vi "1A Interpret NMEA Sentence.vi"(11 "NMEA Sentence":string) -> ()   [LabVIEW 2011]
doc: "Interprets the NMEA 0813 sentences that we are using from our Airmar PB200 WeatherStation sensor.\nBy Jaime McCandless\nTODO: finish implementing NMEA sentences"
uses:
  2-Think/2 Typedefs/Velocity.ctl
  2-Think/2 Typedefs/apparent wind.ctl
  2-Think/2 Typedefs/pitch and roll.ctl
  2-Think/2 Globals/2 Global.vi
  <vilib>/regexp/Match Regular Expression.xnode
panel:
  out "Meteorological Data":T1
  in  "UTC Time Zone":i32=-5
  out "Tab Control":T2(tab)
  out "GPS (GGA) Data":T3
  out "GPS (GLL) Data":T4
  out "UTC Time":timestamp
  out "Local Time":timestamp
  out "Lattitude (ddmm.mmmm)":dbl format="%_8g"
  out "Lattitude North/South":string
  out "Longitude (ddmm.mmmm)":dbl format="%_8g"
  out "Longitude East/West":string
  out "Speed over ground (knots)":dbl format="%_3g"
  out "Course over ground (degrees)":dbl format="%_4g"
  out "Magnetic Variation (degrees)":dbl format="%_4g"
  out "Variation East/West":string
  out "GPS (RMC) Data":T5 {"Course over ground (degrees)" format="%#.6g"; "Speed over ground (knots)" format="%#.6g"; "Magnetic Variation (degrees)" format="%#.6g"; "Longitude (ddmm.mmmm)" format="%#.6g"; "Lattitude (ddmm.mmmm)" format="%#.6g"}
  out "GPS Data Valid?":bool
  out "GPS (VTG) Data":T6
  out "Heading":dbl
  out "Turn (ROT) Data":T7
  out "Wind (MWV) Data":T8
  out "Transducer (XDR) B Data":cluster{"Pitch (deg)":dbl, "Roll (deg)":dbl}
  out "Transducer (XDR) A Data":T9
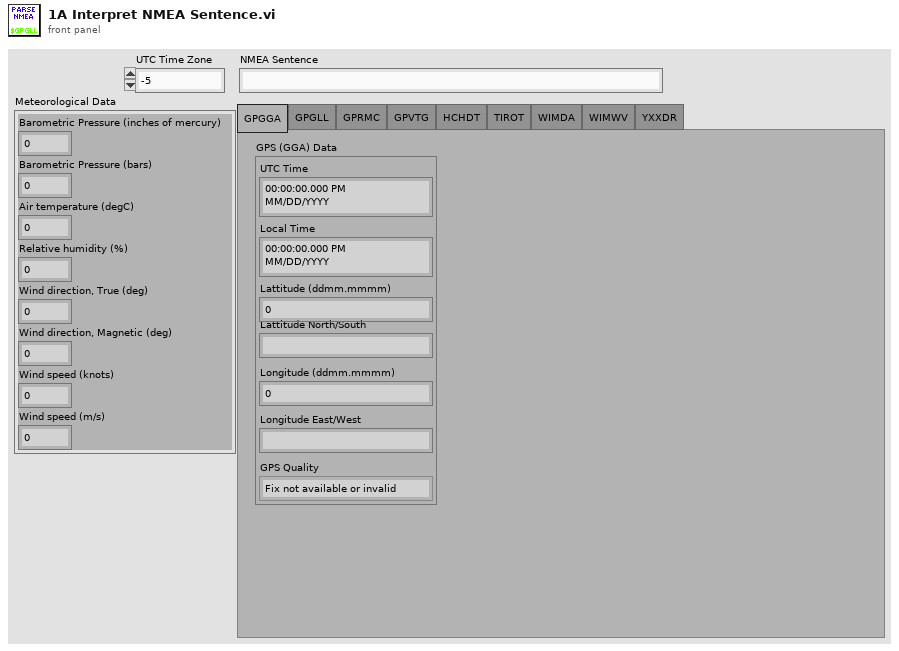
[diagram p1: front panel]
types:
  T1 = cluster{"Barometric Pressure (inches of mercury)":dbl, "Barometric Pressure (bars)":dbl, "Air temperature (degC)":dbl, "Relative humidity (%)":dbl, "Wind direction, True (deg)":dbl, "Wind direction, Magnetic (deg)":dbl, "Wind speed (knots)":dbl, "Wind speed (m/s)":dbl}
  T2 = enum32{"GPGGA", "GPGLL", "GPRMC", "GPVTG", "HCHDT", "TIROT", "WIMDA", "WIMWV", "YXXDR"}
  T3 = cluster{"UTC Time":timestamp, "Local Time":timestamp, "Lattitude (ddmm.mmmm)":dbl, "Lattitude North/South":string, "Longitude (ddmm.mmmm)":dbl, "Longitude East/West":string, "GPS Quality":enum16{"Fix not available or invalid", "GPS SPS Mode, fix valid", "Differential GPS, SPS Mode, fix valid", "GPS PPS Mode, fix valid", "Real Time Kinematic (RTK)", "Float RTK", "Estimated (dead reckoning) Mode", "Manual Input Mode", "Simulator Mode"}}
  T4 = cluster{"UTC Time":timestamp, "Local Time":timestamp, "Lattitude (ddmm.mmmm)":dbl, "Lattitude North/South":string, "Longitude (ddmm.mmmm)":dbl, "Longitude East/West":string, "GPS Mode":string, "GPS Data Valid?":bool}
  T5 = cluster{"UTC Time":timestamp, "Local Time":timestamp, "Lattitude (ddmm.mmmm)":dbl, "Lattitude North/South":string, "Longitude (ddmm.mmmm)":dbl, "Longitude East/West":string, "Magnetic Variation (degrees)":dbl, "Variation East/West":string, "Speed over ground (knots)":dbl, "Course over ground (degrees)":dbl}
  T6 = cluster{"Course Over Ground (True)":dbl, "Course Over Ground (Magnetic)":dbl, "Speed Over Ground (Knots)":dbl, "Speed Over Ground (km/hr)":dbl, "GPS Mode":string}
  T7 = cluster{"Rate of Turn (deg/min)":dbl, "Turn Rotation Data Valid?":bool}
  T8 = cluster{"Angle relative to boat (deg)":dbl, "Wind Data Valid?":bool, "Wind speed (knots)":dbl, "True (T) or Relative (R)":string}
  T9 = cluster{"Calc. Relative Wind Chill (degC)":dbl, "Calc. Theoretical Wind Chill (degC)":dbl, "Calc. Heat Index (degC)":dbl, "Meas. Barometric Pressure (bars)":dbl}
  T10 = cluster{"second":i32, "minute":i32, "hour":i32, "day of month":i32, "month":i32, "year":i32, "day of week":i32, "day of year":i32, "is DST":i32}
  T11 = typedef "Velocity.ctl" = cluster{"East":dbl, "North":dbl}
  T12 = typedef "apparent wind.ctl" = cluster{"Toward Fore":dbl, "Toward Starboard":dbl}
  T13 = typedef "pitch and roll.ctl" = cluster{"Pitch":dbl, "Roll":dbl}
  T14 = typedef "UTM Location.ctl" = cluster{"UTM Zone":dbl, "Hemisphere":enum16{"North", "South"}, "East":dbl, "North":dbl}
  T15 = typedef "generalized sensor status.ctl" = cluster{"Sensor Connected":T16, "Sensor Initialized":T16, "Sensor OK":T16, "Latest Error String":string, "GPS Lock":T16}
  T16 = typedef "indicator LED.ctl" = bool
  T17 = typedef "robot velocity.ctl" = cluster{"East":dbl, "North":dbl}
  T18 = typedef "heading.ctl" = dbl
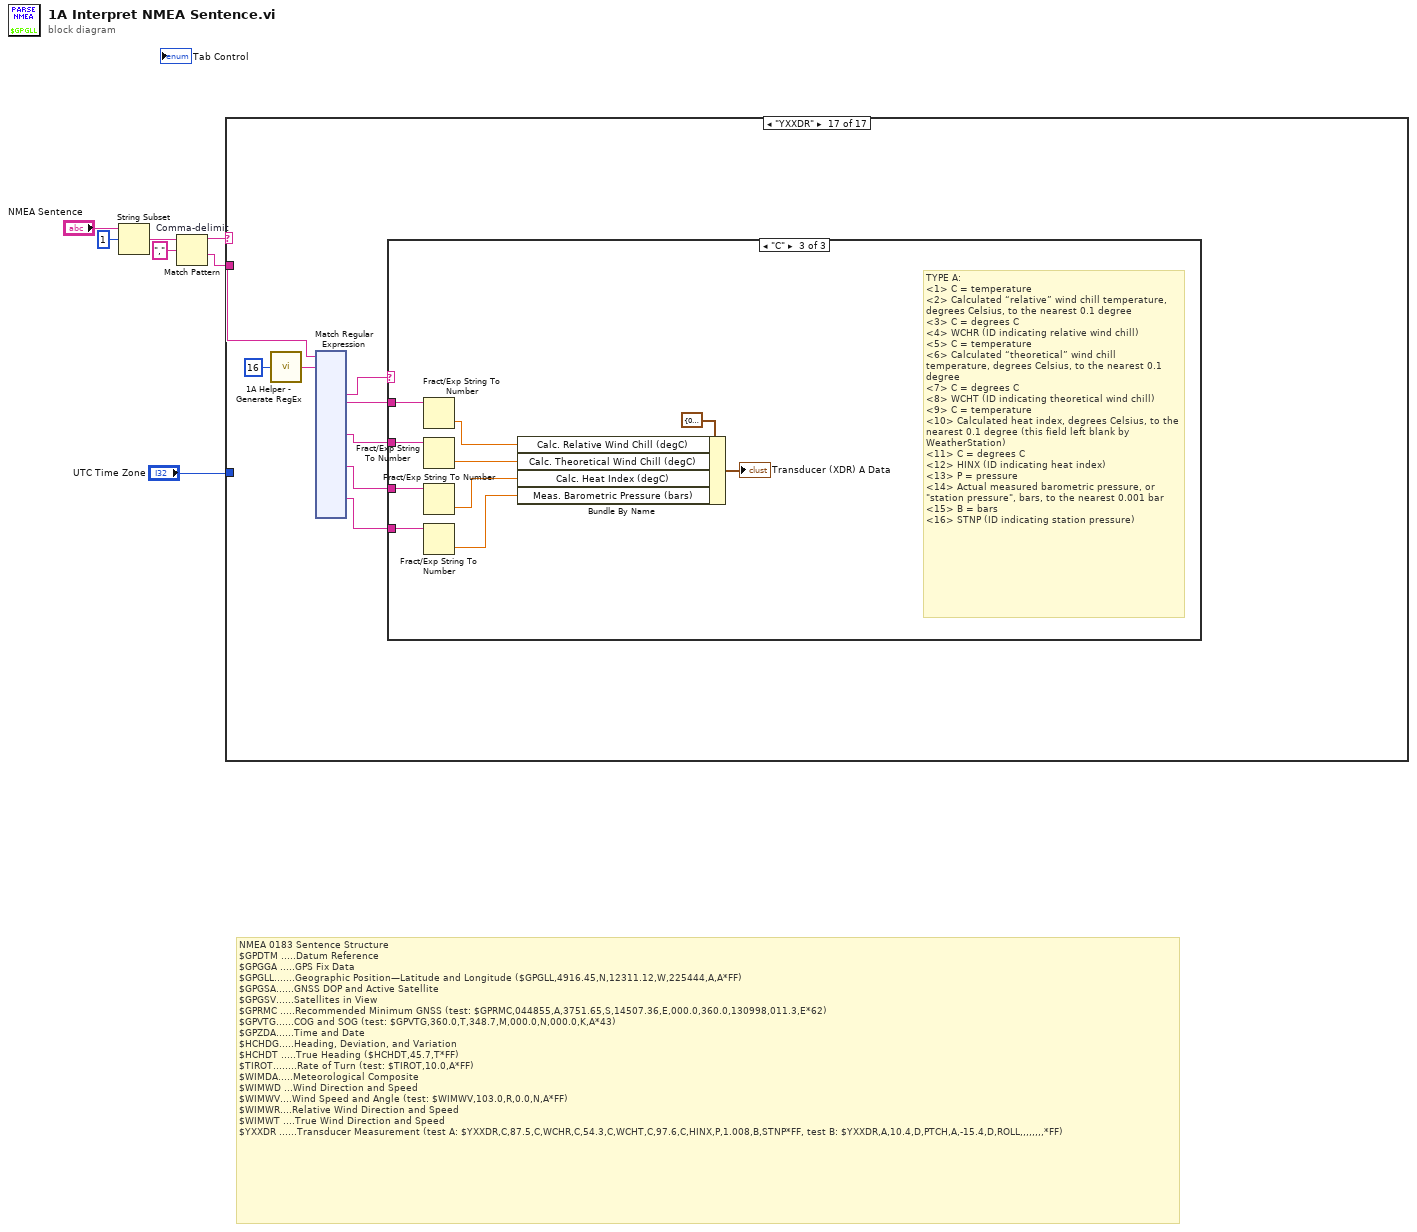
[diagram p0: block diagram]
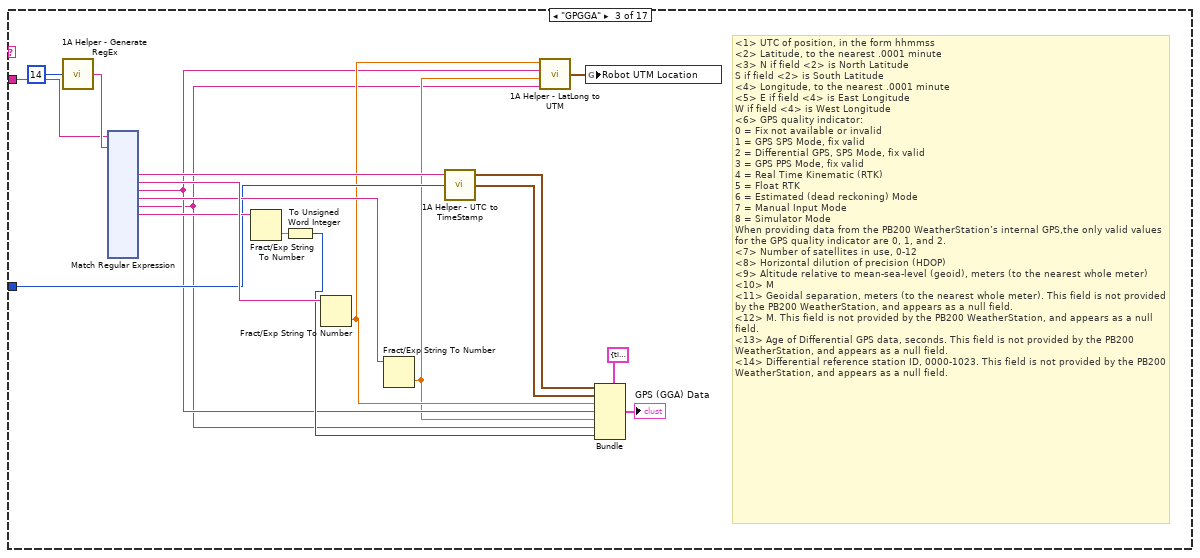
[diagram p4: hidden frame]
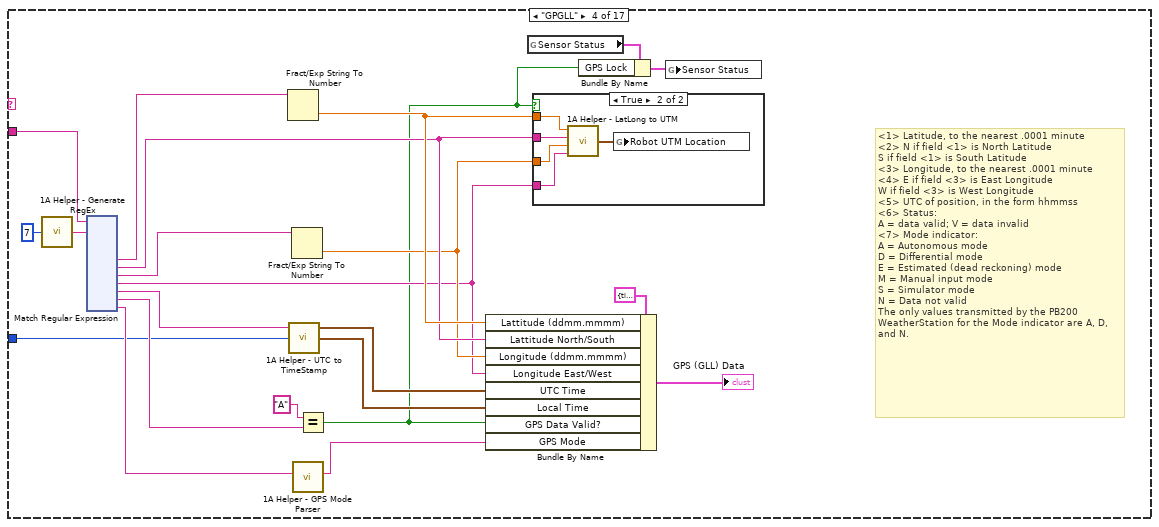
[diagram p5: hidden frame]
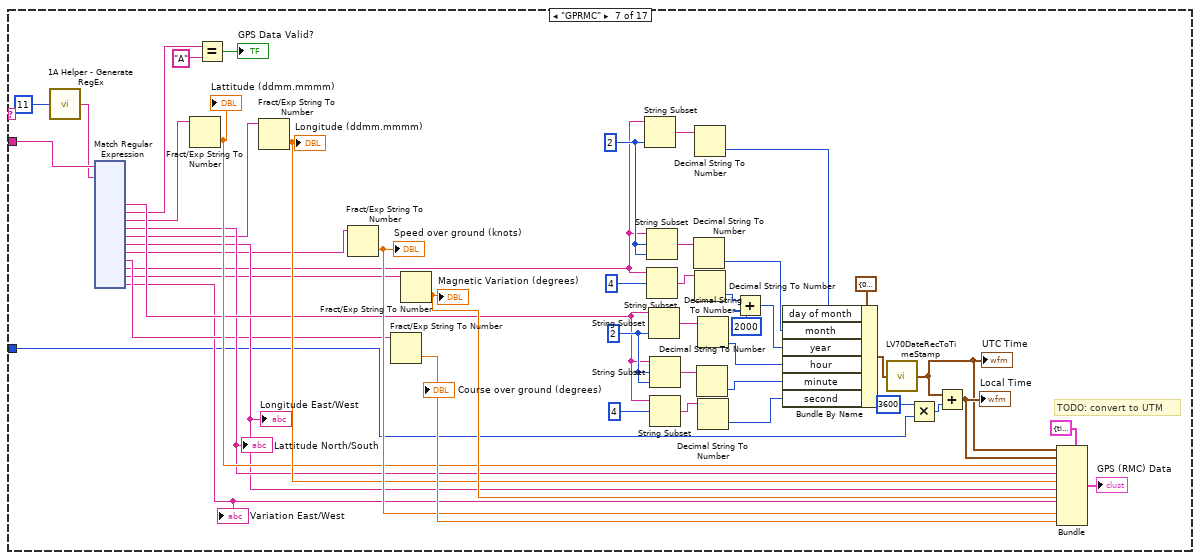
[diagram p9: hidden frame]
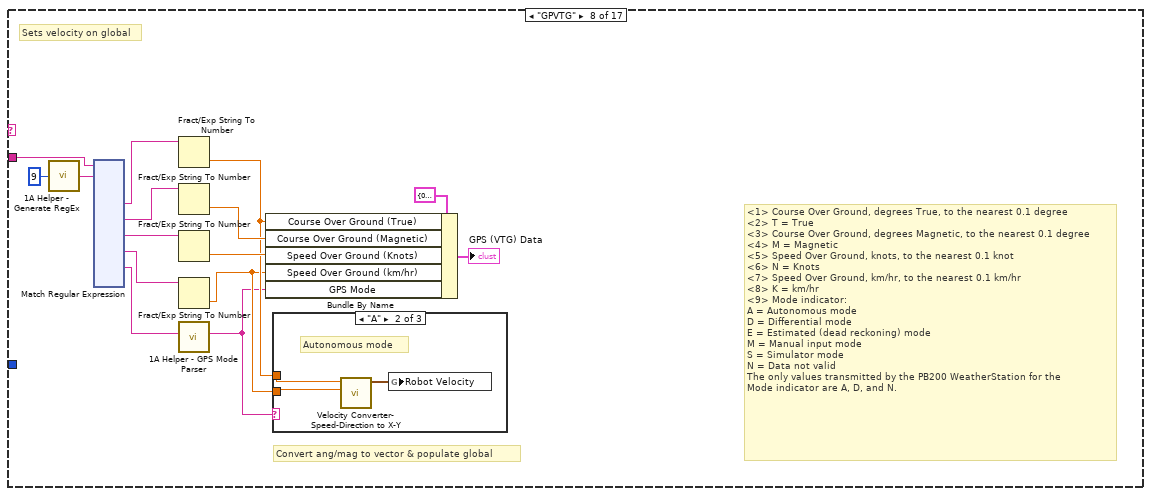
[diagram p10: hidden frame]
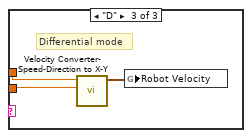
[diagram p12: hidden frame]
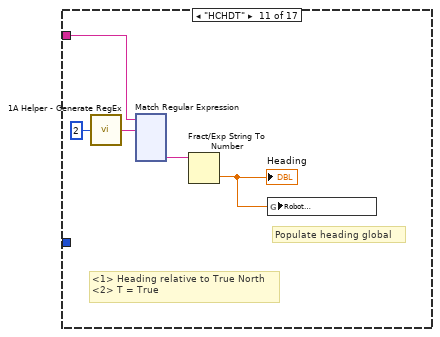
[diagram p15: hidden frame]
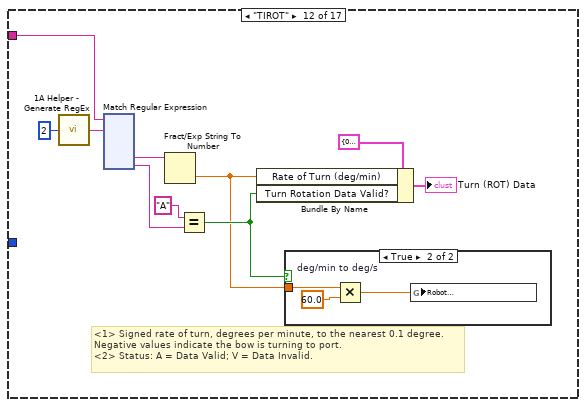
[diagram p16: hidden frame]
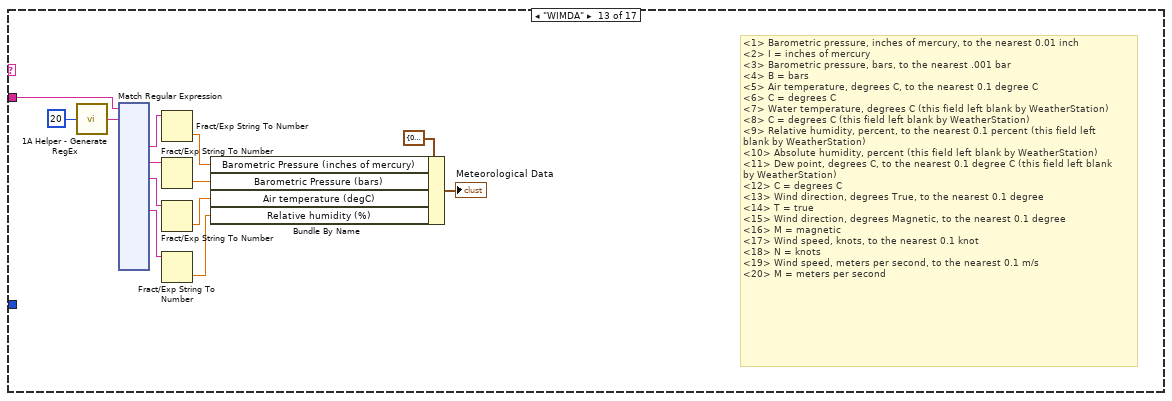
[diagram p18: hidden frame]
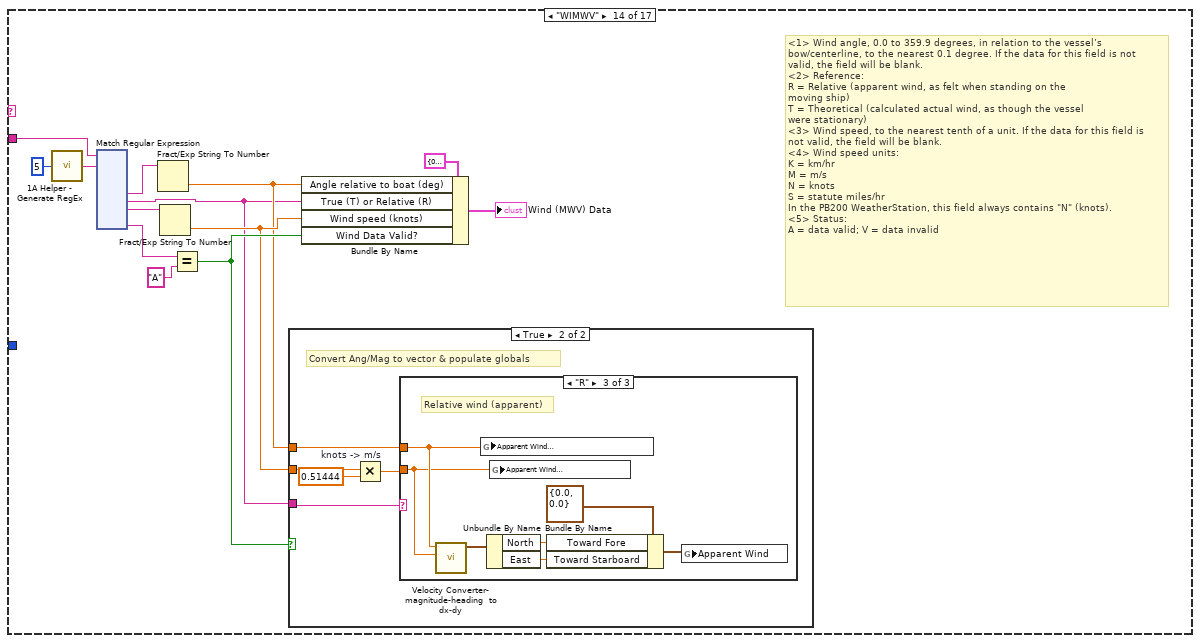
[diagram p19: hidden frame]
diagram:
  # "NMEA 0183 Sentence Structure\n$GPDTM .....Datum Reference\n$GPGGA .....GPS Fix Data\n$GPGLL.......Geographic Position—Latitude and Longitude ($GPGLL,4916.45,N,12311.12,W,225444,A,A*FF)\n$GPGSA......GNSS DOP and Active Satellite\n$GPGSV......Satellites in View\n$GPRMC .....Recommended Minimum GNSS (test: $GPRMC,044855,A,3751.65,S,14507.36,E,000.0,360.0,130998,011.3,E*62)\n$GPVTG......COG and SOG (test: $GPVTG,360.0,T,348.7,M,000.0,N,000.0,K,A*43)\n$GPZDA......Time and Date\n$HCHDG.....Heading, Deviation, and Variation\n$HCHDT .....True Heading ($HCHDT,45.7,T*FF)\n$TIROT........Rate of Turn (test: $TIROT,10.0,A*FF)\n$WIMDA.....Meteorological Composite\n$WIMWD ...Wind Direction and Speed\n$WIMWV....Wind Speed and Angle (test: $WIMWV,103.0,R,0.0,N,A*FF)\n$WIMWR....Relative Wind Direction and Speed\n$WIMWT ....True Wind Direction and Speed\n$YXXDR ......Transducer Measurement (test A: $YXXDR,C,87.5,C,WCHR,C,54.3,C,WCHT,C,97.6,C,HINX,P,1.008,B,STNP*FF, test B: $YXXDR,A,10.4,D,PTCH,A,-15.4,D,ROLL,,,,,,,,*FF)"
  n1 = String Subset(string="NMEA Sentence", offset (0)=1) -> (substring=w4:string)  [unwired: 1 in]
  n2 = Match Pattern "Comma-delimit"(string=w4, regular expression=",") -> (before substring=w5:string, after substring=w6:string)  [unwired: 1 in, 2 out]
  n3 = case shown="\"YXXDR\"" w5 {
    tunnel: w6 -> [_ _ w24 w166 _ _ w310 w479 _ _ w613 w735 w866 w1005 _ _ w1153]
    tunnel: "UTC Time Zone" -> [_ _ w13 w158 _ _ w296 _ _ _ _ _ _ _ _ _ _]
    frame "", Default {
    }
    frame "GPDTM" {
      # "unimplemented"
    }
    frame "GPGGA" {
      # "<1> UTC of position, in the form hhmmss\n<2> Latitude, to the nearest .0001 minute\n<3> N if field <2> is North Latitude\nS if field <2> is South Latitude\n<4> Longitude, to the nearest .0001 minute\n<5> E if field <4> is East Longitude\nW if field <4> is West Longitude\n<6> GPS quality indicator:\n0 = Fix not available or invalid\n1 = GPS SPS Mode, fix valid\n2 = Differential GPS, SPS Mode, fix valid\n3 = GPS PPS Mode, fix valid\n4 = Real Time Kinematic (RTK)\n5 = Float RTK\n6 = Estimated (dead reckoning) Mode\n7 = Manual Input Mode\n8 = Simulator Mode\nWhen providing data from the PB200 WeatherStation’s internal GPS,the only valid values for the GPS quality indicator are 0, 1, and 2.\n<7> Number of satellites in use, 0-12\n<8> Horizontal dilution of precision (HDOP)\n<9> Altitude relative to mean-sea-level (geoid), meters (to the nearest whole meter)\n<10> M\n<11> Geoidal separation, meters (to the nearest whole meter). This field is not provided by the PB200 WeatherStation, and appears as a null field.\n<12> M. This field is not provided by the PB200 WeatherStation, and appears as a null field.\n<13> Age of Differential GPS data, seconds. This field is not provided by the PB200 WeatherStation, and appears as a null field.\n<14> Differential reference station ID, 0000-1023. This field is not provided by the PB200 WeatherStation, and appears as a null field."
      n4 = call "1A Helper - Generate RegEx.vi"("# Datums"=14) -> ("RegEx"=w25:string)
      n5 = xnode "Match Regular Expression"("input string"=w24, "regular expression"=w25) -> ("submatch 1"=w16:string, "submatch 2"=w22:string, "submatch 3"=w10:string, "submatch 4"=w21:string, "submatch 5"=w8:string, "submatch 6"=w20:string)  [unwired: 4 in, 10 out]
      n6 = Fract/Exp String To Number(string=w20) -> (number=w19:dbl)  [unwired: 3 in, 1 out]
      n7 = To Unsigned Word Integer(number=w19) -> (unsigned 16bit integer=w18:u16)
      n8 = Fract/Exp String To Number(string=w22) -> (number=w11:dbl)  [unwired: 3 in, 1 out]
      n9 = Fract/Exp String To Number(string=w21) -> (number=w9:dbl)  [unwired: 3 in, 1 out]
      n10 = call "1A Helper - UTC to TimeStamp.vi"("UTC Time Zone in"=w13, "UTC (hhmmss)"=w16) -> ("Local Time"=w14:timestamp, "UTC Time"=w15:timestamp)  [unwired: 2 in]
      n11 = call "1A Helper - LatLong to UTM.vi"("East/West"=w8, "Longitude"=w9, "North/South"=w10, "Latitude"=w11) -> ("Robot UTM Location"=w12:T14)
      n12 = global write "2 Global.vi" "Robot UTM Location"(w12) -> ()
      n13 = Bundle(cluster=T3 {"UTC Time"=timestamp(0 s since 1904-01-01), "Local Time"=timestamp(0 s since 1904-01-01), "Lattitude (ddmm.mmmm)"=0.0, "Lattitude North/South"="", "Longitude (ddmm.mmmm)"=0.0, "Longitude East/West"="", "GPS Quality"=enum."GPS SPS Mode, fix valid"} ("Cluster"), "UTC Time"=w15, "Local Time"=w14, "Lattitude (ddmm.mmmm)"=w11, "Lattitude North/South"=w10, "Longitude (ddmm.mmmm)"=w9, "Longitude East/West"=w8, "GPS Quality"=w18) -> (→"GPS (GGA) Data":T3)
    }
    frame "GPGLL" {
      # "<1> Latitude, to the nearest .0001 minute\n<2> N if field <1> is North Latitude\nS if field <1> is South Latitude\n<3> Longitude, to the nearest .0001 minute\n<4> E if field <3> is East Longitude\nW if field <3> is West Longitude\n<5> UTC of position, in the form hhmmss\n<6> Status:\nA = data valid; V = data invalid\n<7> Mode indicator:\nA = Autonomous mode\nD = Differential mode\nE = Estimated (dead reckoning) mode\nM = Manual input mode\nS = Simulator mode\nN = Data not valid\nThe only values transmitted by the PB200 WeatherStation for the Mode indicator are A, D, and N."
      n14 = call "1A Helper - Generate RegEx.vi"("# Datums"=7) -> ("RegEx"=w170:string)
      n15 = xnode "Match Regular Expression"("input string"=w166, "regular expression"=w170) -> ("submatch 1"=w169:string, "submatch 2"=w155:string, "submatch 3"=w168:string, "submatch 4"=w153:string, "submatch 5"=w165:string, "submatch 6"=w161:string, "submatch 7"=w167:string)  [unwired: 4 in, 5 out]
      n16 = Fract/Exp String To Number(string=w169) -> (number=w156:dbl)  [unwired: 3 in, 1 out]
      n17 = call "1A Helper - UTC to TimeStamp.vi"("UTC Time Zone in"=w158, "UTC (hhmmss)"=w165) -> ("Local Time"=w160:timestamp, "UTC Time"=w159:timestamp)  [unwired: 2 in]
      n18 = Fract/Exp String To Number(string=w168) -> (number=w154:dbl)  [unwired: 3 in, 1 out]
      n19 = call "1A Helper - GPS Mode Parser.vi"("GPS Mode (Char)"=w167) -> ("GPS Mode (Description)"=w163:string)  [unwired: 6 in]
      n20 = Equal?(x="A" ("y"), y=w161) -> (x = y?=w150:bool)
      n21 = Bundle By Name(cluster=T4 {"UTC Time"=timestamp(0 s since 1904-01-01), "Local Time"=timestamp(0 s since 1904-01-01), "Lattitude (ddmm.mmmm)"=0.0, "Lattitude North/South"="", "Longitude (ddmm.mmmm)"=0.0, "Longitude East/West"="", "GPS Mode"="", "GPS Data Valid?"=FALSE} ("Cluster"), "Lattitude (ddmm.mmmm)"=w156, "Lattitude North/South"=w155, "Longitude (ddmm.mmmm)"=w154, "Longitude East/West"=w153, "UTC Time"=w159, "Local Time"=w160, "GPS Data Valid?"=w150, "GPS Mode"=w163) -> (→"GPS (GLL) Data":T4)
      n22 = global read "2 Global.vi" "Sensor Status"() -> (w151:T15)
      n23 = case shown="True" w150 {
        tunnel: w156 -> [_ w176]
        tunnel: w155 -> [_ w175]
        tunnel: w154 -> [_ w174]
        tunnel: w153 -> [_ w173]
        frame False {
        }
        frame True {
          n24 = call "1A Helper - LatLong to UTM.vi"("East/West"=w173, "Longitude"=w174, "North/South"=w175, "Latitude"=w176) -> ("Robot UTM Location"=w172:T14)
          n25 = global write "2 Global.vi" "Robot UTM Location"(w172) -> ()
        }
      }
      n26 = Bundle By Name(cluster=w151, "GPS Lock"=w150) -> (w152:T15)
      n27 = global write "2 Global.vi" "Sensor Status"(w152) -> ()
    }
    frame "GPGSA" {
      # "unimplemented"
    }
    frame "GPGSV" {
      # "unimplemented"
    }
    frame "GPRMC" {
      w328 = 2 ("length (rest)")
      w318 = 2 ("length (rest)")
      # "TODO: convert to UTM"
      n28 = call "1A Helper - Generate RegEx.vi"("# Datums"=11) -> ("RegEx"=w298:string)
      n29 = xnode "Match Regular Expression"("input string"=w310, "regular expression"=w298) -> ("submatch 1"=w309:string, "submatch 2"=w308:string, "submatch 3"=w307:string, "submatch 4"=w306:string, "submatch 5"=w305:string, "submatch 6"=w304:string, "submatch 7"=w303:string, "submatch 8"=w302:string, "submatch 9"=w301:string, "submatch 10"=w300:string, "submatch 11"=w299:string)  [unwired: 4 in, 5 out]
      "Lattitude North/South" <- w306
      "Longitude East/West" <- w304
      "Variation East/West" <- w299
      n30 = Fract/Exp String To Number(string=w307) -> (number=w337:dbl)  [unwired: 3 in, 1 out]
      "Lattitude (ddmm.mmmm)" <- w337
      n31 = Equal?(x=w308, y="A") -> (x = y?=→"GPS Data Valid?":bool)
      n32 = Fract/Exp String To Number(string=w305) -> (number=w338:dbl)  [unwired: 3 in, 1 out]
      "Longitude (ddmm.mmmm)" <- w338
      n33 = Fract/Exp String To Number(string=w303) -> (number=w340:dbl)  [unwired: 3 in, 1 out]
      "Speed over ground (knots)" <- w340
      n34 = Fract/Exp String To Number(string=w302) -> (number=w341:dbl)  [unwired: 3 in, 1 out]
      "Course over ground (degrees)" <- w341
      n35 = Fract/Exp String To Number(string=w300) -> (number=w339:dbl)  [unwired: 3 in, 1 out]
      "Magnetic Variation (degrees)" <- w339
      n36 = String Subset(string=w301, length (rest)=w328) -> (substring=w329:string)  [unwired: 1 in]
      n37 = String Subset(string=w301, offset (0)=w328, length (rest)=w328) -> (substring=w327:string)
      n38 = String Subset(string=w301, offset (0)=4) -> (substring=w325:string)  [unwired: 1 in]
      n39 = String Subset(string=w309, length (rest)=w318) -> (substring=w314:string)  [unwired: 1 in]
      n40 = String Subset(string=w309, offset (0)=w318, length (rest)=w318) -> (substring=w320:string)
      n41 = String Subset(string=w309, offset (0)=4) -> (substring=w322:string)  [unwired: 1 in]
      n42 = Decimal String To Number(string=w327) -> (number=w331:i32)  [unwired: 2 in, 1 out]
      n43 = Decimal String To Number(string=w329) -> (number=w330:i32)  [unwired: 2 in, 1 out]
      n44 = Decimal String To Number(string=w325) -> (number=w332:i32)  [unwired: 2 in, 1 out]
      n45 = Decimal String To Number(string=w320) -> (number=w319:i32)  [unwired: 2 in, 1 out]
      n46 = Decimal String To Number(string=w314) -> (number=w317:i32)  [unwired: 2 in, 1 out]
      n47 = Decimal String To Number(string=w322) -> (number=w323:i32)  [unwired: 2 in, 1 out]
      n48 = Add(x=w332, y=2000) -> (x+y=w334:i32)
      n49 = Bundle By Name(cluster=T10 {"second"=0, "minute"=0, "hour"=0, "day of month"=0, "month"=0, "year"=0, "day of week"=0, "day of year"=0, "is DST"=0} ("date time rec"), "day of month"=w330, "month"=w331, "year"=w334, "hour"=w317, "minute"=w319, "second"=w323) -> (w315:T10)
      n50 = call <vilib>:"LV70DateRecToTimeStamp.vi"("date time rec"=w315) -> ("Time Stamp"=w335:timestamp)
      "UTC Time" <- w335
      n51 = Multiply(x=3600 ("number"), y=w296) -> (x*y=w297:i32)
      n52 = Add(x=w335, y=w297) -> (x+y=w336:timestamp)
      "Local Time" <- w336
      n53 = Bundle(cluster=T5 {"UTC Time"=timestamp(0 s since 1904-01-01), "Local Time"=timestamp(0 s since 1904-01-01), "Lattitude (ddmm.mmmm)"=0.0, "Lattitude North/South"="", "Longitude (ddmm.mmmm)"=0.0, "Longitude East/West"="", "Magnetic Variation (degrees)"=0.0, "Variation East/West"="", "Speed over ground (knots)"=0.0, "Course over ground (degrees)"=0.0} ("Cluster"), "UTC Time"=w335, "Local Time"=w336, "Lattitude (ddmm.mmmm)"=w337, "Lattitude North/South"=w306, "Longitude (ddmm.mmmm)"=w338, "Longitude East/West"=w304, "Magnetic Variation (degrees)"=w339, "Variation East/West"=w299, "Speed over ground (knots)"=w340, "Course over ground (degrees)"=w341) -> (→"GPS (RMC) Data":T5)
    }
    frame "GPVTG" {
      # "Convert ang/mag to vector & populate global"
      # "Sets velocity on global"
      # "<1> Course Over Ground, degrees True, to the nearest 0.1 degree\n<2> T = True\n<3> Course Over Ground, degrees Magnetic, to the nearest 0.1 degree\n<4> M = Magnetic\n<5> Speed Over Ground, knots, to the nearest 0.1 knot\n<6> N = Knots\n<7> Speed Over Ground, km/hr, to the nearest 0.1 km/hr\n<8> K = km/hr\n<9> Mode indicator:\nA = Autonomous mode\nD = Differential mode\nE = Estimated (dead reckoning) mode\nM = Manual input mode\nS = Simulator mode\nN = Data not valid\nThe only values transmitted by the PB200 WeatherStation for the\nMode indicator are A, D, and N."
      n54 = call "1A Helper - Generate RegEx.vi"("# Datums"=9) -> ("RegEx"=w480:string)
      n55 = xnode "Match Regular Expression"("input string"=w479, "regular expression"=w480) -> ("submatch 1"=w476:string, "submatch 3"=w475:string, "submatch 5"=w473:string, "submatch 7"=w471:string, "submatch 9"=w470:string)  [unwired: 4 in, 11 out]
      n56 = Fract/Exp String To Number(string=w476) -> (number=w469:dbl)  [unwired: 3 in, 1 out]
      n57 = Fract/Exp String To Number(string=w475) -> (number=w474:dbl)  [unwired: 3 in, 1 out]
      n58 = Fract/Exp String To Number(string=w473) -> (number=w472:dbl)  [unwired: 3 in, 1 out]
      n59 = Fract/Exp String To Number(string=w471) -> (number=w468:dbl)  [unwired: 3 in, 1 out]
      n60 = call "1A Helper - GPS Mode Parser.vi"("GPS Mode (Char)"=w470) -> ("GPS Mode (Description)"=w467:string)  [unwired: 6 in]
      n61 = Bundle By Name(cluster=T6 {"Course Over Ground (True)"=0.0, "Course Over Ground (Magnetic)"=0.0, "Speed Over Ground (Knots)"=0.0, "Speed Over Ground (km/hr)"=0.0, "GPS Mode"=""} ("GPS (VTG) Data 2"), "Course Over Ground (True)"=w469, "Course Over Ground (Magnetic)"=w474, "Speed Over Ground (Knots)"=w472, "Speed Over Ground (km/hr)"=w468, "GPS Mode"=w467) -> (→"GPS (VTG) Data":T6)
      n62 = case shown="\"A\"" w467 {
        tunnel: w469 -> [_ w482 w487]
        tunnel: w468 -> [_ w484 w486]
        frame "N", Default {
          # "Data not valid"
        }
        frame "A" {
          # "Autonomous mode"
          n63 = call "Velocity Converter- Speed-Direction to X-Y.vi"("Speed"=w484, "Heading"=w482) -> ("Robot Velocity Out"=w483:T17)  [unwired: 9 in]
          n64 = global write "2 Global.vi" "Robot Velocity"(w483) -> ()
        }
        frame "D" {
          # "Differential mode"
          n65 = call "Velocity Converter- Speed-Direction to X-Y.vi"("Speed"=w486, "Heading"=w487) -> ("Robot Velocity Out"=w485:T17)  [unwired: 9 in]
          n66 = global write "2 Global.vi" "Robot Velocity"(w485) -> ()
        }
      }
    }
    frame "GPZDA" {
      # "<1> UTC time of day, in the form hhmmss\n<2> UTC day, 01 to 31\n<3> UTC month, 01 to 12\n<4> UTC year (four digits, e.g. 2006)\n<5> Local time zone hours, 00 to +/-13 hrs\n<6> Local time zone minutes, 00 to +59"
    }
    frame "HCHDG " {
      # "<1> Magnetic sensor heading, degrees, to the nearest 0.1 degree.\n<2> Magnetic deviation, degrees east or west, to the nearest 0.1 degree.\n<3> E if field <2> is degrees East\nW if field <2> is degrees West\n<4> Magnetic variation, degrees east or west, to the nearest 0.1 degree.\n<5> E if field <4> is degrees East\nW if field <4> is degrees West"
    }
    frame "HCHDT" {
      # "Populate heading global"
      # "<1> Heading relative to True North\n<2> T = True"
      n67 = call "1A Helper - Generate RegEx.vi"("# Datums"=2) -> ("RegEx"=w614:string)
      n68 = xnode "Match Regular Expression"("input string"=w613, "regular expression"=w614) -> ("submatch 1"=w612:string)  [unwired: 4 in, 5 out]
      n69 = Fract/Exp String To Number(string=w612) -> (number=w611:dbl)  [unwired: 3 in, 1 out]
      "Heading" <- w611
      n70 = global write "2 Global.vi" "Robot\nHeading"(w611) -> ()
    }
    frame "TIROT" {
      # "<1> Signed rate of turn, degrees per minute, to the nearest 0.1 degree.\nNegative values indicate the bow is turning to port.\n<2> Status: A = Data Valid; V = Data Invalid."
      n71 = call "1A Helper - Generate RegEx.vi"("# Datums"=2) -> ("RegEx"=w737:string)
      n72 = xnode "Match Regular Expression"("input string"=w735, "regular expression"=w737) -> ("submatch 1"=w736:string, "submatch 2"=w731:string)  [unwired: 4 in, 5 out]
      n73 = Fract/Exp String To Number(string=w736) -> (number=w729:dbl)  [unwired: 3 in, 1 out]
      n74 = Equal?(x="A" ("y"), y=w731) -> (x = y?=w730:bool)
      n75 = Bundle By Name(cluster=T7 {"Rate of Turn (deg/min)"=0.0, "Turn Rotation Data Valid?"=TRUE} ("Turn (ROT) Data 2"), "Rate of Turn (deg/min)"=w729, "Turn Rotation Data Valid?"=w730) -> (→"Turn (ROT) Data":T7)
      n76 = case shown="True" w730 {
        tunnel: w729 -> [_ w740]
        frame False {
        }
        frame True {
          n77 = Multiply "deg/min to deg/s"(x=w740, y=60.0) -> (x*y=w741:dbl)
          n78 = global write "2 Global.vi" "Robot\nRate of Turn"(w741) -> ()
        }
      }
    }
    frame "WIMDA" {
      # "<1> Barometric pressure, inches of mercury, to the nearest 0.01 inch\n<2> I = inches of mercury\n<3> Barometric pressure, bars, to the nearest .001 bar\n<4> B = bars\n<5> Air temperature, degrees C, to the nearest 0.1 degree C\n<6> C = degrees C\n<7> Water temperature, degrees C (this field left blank by WeatherStation)\n<8> C = degrees C (this field left blank by WeatherStation)\n<9> Relative humidity, percent, to the nearest 0.1 percent (this field left\nblank by WeatherStation)\n<10> Absolute humidity, percent (this field left blank by WeatherStation)\n<11> Dew point, degrees C, to the nearest 0.1 degree C (this field left blank\nby WeatherStation)\n<12> C = degrees C\n<13> Wind direction, degrees True, to the nearest 0.1 degree\n<14> T = true\n<15> Wind direction, degrees Magnetic, to the nearest 0.1 degree\n<16> M = magnetic\n<17> Wind speed, knots, to the nearest 0.1 knot\n<18> N = knots\n<19> Wind speed, meters per second, to the nearest 0.1 m/s\n<20> M = meters per second"
      n79 = call "1A Helper - Generate RegEx.vi"("# Datums"=20) -> ("RegEx"=w867:string)
      n80 = xnode "Match Regular Expression"("input string"=w866, "regular expression"=w867) -> ("submatch 1"=w860:string, "submatch 3"=w859:string, "submatch 5"=w858:string, "submatch 9"=w857:string)  [unwired: 4 in, 17 out]
      n81 = Fract/Exp String To Number(string=w860) -> (number=w864:dbl)  [unwired: 3 in, 1 out]
      n82 = Fract/Exp String To Number(string=w859) -> (number=w863:dbl)  [unwired: 3 in, 1 out]
      n83 = Fract/Exp String To Number(string=w858) -> (number=w862:dbl)  [unwired: 3 in, 1 out]
      n84 = Fract/Exp String To Number(string=w857) -> (number=w861:dbl)  [unwired: 3 in, 1 out]
      n85 = Bundle By Name(cluster=T1 {"Barometric Pressure (inches of mercury)"=0.0, "Barometric Pressure (bars)"=0.0, "Air temperature (degC)"=0.0, "Relative humidity (%)"=0.0, "Wind direction, True (deg)"=0.0, "Wind direction, Magnetic (deg)"=0.0, "Wind speed (knots)"=0.0, "Wind speed (m/s)"=0.0} ("Meteorological Data"), "Barometric Pressure (inches of mercury)"=w864, "Barometric Pressure (bars)"=w863, "Air temperature (degC)"=w862, "Relative humidity (%)"=w861) -> (→"Meteorological Data":T1)
    }
    frame "WIMWV" {
      # "<1> Wind angle, 0.0 to 359.9 degrees, in relation to the vessel’s\nbow/centerline, to the nearest 0.1 degree. If the data for this field is not\nvalid, the field will be blank.\n<2> Reference:\nR = Relative (apparent wind, as felt when standing on the\nmoving ship)\nT = Theoretical (calculated actual wind, as though the vessel\nwere stationary)\n<3> Wind speed, to the nearest tenth of a unit. If the data for this field is\nnot valid, the field will be blank.\n<4> Wind speed units:\nK = km/hr\nM = m/s\nN = knots\nS = statute miles/hr\nIn the PB200 WeatherStation, this field always contains \"N\" (knots).\n<5> Status:\nA = data valid; V = data invalid"
      n86 = call "1A Helper - Generate RegEx.vi"("# Datums"=5) -> ("RegEx"=w1008:string)
      n87 = xnode "Match Regular Expression"("input string"=w1005, "regular expression"=w1008) -> ("submatch 1"=w1007:string, "submatch 2"=w997:string, "submatch 3"=w1002:string, "submatch 5"=w1001:string)  [unwired: 4 in, 6 out]
      n88 = Fract/Exp String To Number(string=w1007) -> (number=w998:dbl)  [unwired: 3 in, 1 out]
      n89 = Fract/Exp String To Number(string=w1002) -> (number=w999:dbl)  [unwired: 3 in, 1 out]
      n90 = Equal?(x=w1001, y="A") -> (x = y?=w1000:bool)
      n91 = case shown="True" w1000 {
        tunnel: w999 -> [_ w1011]
        tunnel: w998 -> [_ w1014]
        tunnel: w997 -> [_ w1013]
        frame False {
        }
        frame True {
          # "Convert Ang/Mag to vector & populate globals"
          n92 = Multiply "knots -> m/s"(x=w1011, y=0.51444) -> (x*y=w1012:dbl)
          n93 = case shown="\"R\"" w1013 {
            tunnel: w1012 -> [_ w1019 w1024]
            tunnel: w1014 -> [_ w1016 w1025]
            frame "", Default {
            }
            frame "T" {
              # "Theoretical wind (absolute)"
              n94 = global read "2 Global.vi" "Robot\nHeading"() -> (w1017:T18)
              n95 = Add "Get relative to compass, not boat"(x=w1017, y=w1016) -> (x+y=w1015:T18)
              n96 = call "Velocity Converter- magnitude-heading  to dx-dy.vi"("Magnitude"=w1019, "Heading"=w1015) -> ("Vector Out"=w1023:T11)  [unwired: 9 in]
              n97 = Unbundle By Name(w1023) -> ("North"=w1021:dbl, "East"=w1020:dbl)
              n98 = Bundle By Name(cluster=T11 {"East"=0.0, "North"=0.0} ("Absolute Wind"), "North"=w1021, "East"=w1020) -> (w1022:T11)
              n99 = global write "2 Global.vi" "Absolute Wind\nDirection (º)"(w1015) -> ()
              n100 = global write "2 Global.vi" "Absolute Wind\nSpeed"(w1019) -> ()
              n101 = global write "2 Global.vi" "Absolute Wind"(w1022) -> ()
            }
            frame "R" {
              # "Relative wind (apparent)"
              n102 = call "Velocity Converter- magnitude-heading  to dx-dy.vi"("Magnitude"=w1024, "Heading"=w1025) -> ("Vector Out"=w1026:T11)  [unwired: 9 in]
              n103 = global write "2 Global.vi" "Apparent Wind\nDirection (º)"(w1025) -> ()
              n104 = Unbundle By Name(w1026) -> ("North"=w1029:dbl, "East"=w1030:dbl)
              n105 = global write "2 Global.vi" "Apparent Wind\nSpeed"(w1024) -> ()
              n106 = Bundle By Name(cluster=T12 {"Toward Fore"=0.0, "Toward Starboard"=0.0} ("Apparent Wind"), "Toward Fore"=w1029, "Toward Starboard"=w1030) -> (w1028:T12)
              n107 = global write "2 Global.vi" "Apparent Wind"(w1028) -> ()
            }
          }
        }
      }
      n108 = Bundle By Name(cluster=T8 {"Angle relative to boat (deg)"=0.0, "Wind Data Valid?"=TRUE, "Wind speed (knots)"=0.0, "True (T) or Relative (R)"=""} ("Wind (MWV) Data 2"), "Angle relative to boat (deg)"=w998, "True (T) or Relative (R)"=w997, "Wind speed (knots)"=w999, "Wind Data Valid?"=w1000) -> (→"Wind (MWV) Data":T8)
    }
    frame "WIMWR" {
    }
    frame "WIMWT" {
    }
    frame "YXXDR" {
      n109 = call "1A Helper - Generate RegEx.vi"("# Datums"=16) -> ("RegEx"=w1155:string)
      n110 = xnode "Match Regular Expression"("input string"=w1153, "regular expression"=w1155) -> ("submatch 1"=w1152:string, "submatch 2"=w1151:string, "submatch 6"=w1150:string, "submatch 10"=w1149:string, "submatch 14"=w1148:string)  [unwired: 4 in, 16 out]
      n111 = case shown="\"C\"" w1152 {
        tunnel: w1151 -> [_ w1161 w1171]
        tunnel: w1150 -> [_ w1160 w1170]
        tunnel: w1149 -> [_ _ w1168]
        tunnel: w1148 -> [_ _ w1169]
        frame "", Default {
        }
        frame "A" {
          # "TYPE B:\n<1> A = angular displacement\n<2> Pitch: oscillation of vessel about its latitudinal axis. Bow moving up is positive. Value reported to the nearest 0.1 degree.\n<3> D = degrees\n<4> PTCH (ID indicating pitch of vessel)\n<5> A = angular displacement\n<6> Roll: oscillation of vessel about its longitudinal axis. Roll to the starboard is positive. Value reported to the nearest 0.1 degree.\n<7> D = degrees\n<8> ROLL (ID indicating roll of vessel)\n<9> Not used\n<10> Not used\n<11> Not used\n<12> Not used\n<13> Not used\n<14> Not used\n<15> Not used\n<16> Not used"
          n112 = Fract/Exp String To Number(string=w1161) -> (number=w1157:dbl)  [unwired: 3 in, 1 out]
          n113 = Fract/Exp String To Number(string=w1160) -> (number=w1156:dbl)  [unwired: 3 in, 1 out]
          n114 = Bundle By Name(cluster=cluster{"Pitch (deg)":dbl, "Roll (deg)":dbl} {"Pitch (deg)"=103.0, "Roll (deg)"=103.0} ("Transducer (XDR) B Data 2"), "Pitch (deg)"=w1157, "Roll (deg)"=w1156) -> (→"Transducer (XDR) B Data":cluster{"Pitch (deg)":dbl, "Roll (deg)":dbl})
          n115 = Bundle By Name(cluster=T13 {"Pitch"=0.0, "Roll"=0.0} ("Robot Pitch/Roll"), "Pitch"=w1157, "Roll"=w1156) -> (w1158:T13)
          n116 = global write "2 Global.vi" "Robot Pitch/Roll"(w1158) -> ()
        }
        frame "C" {
          # "TYPE A:\n<1> C = temperature\n<2> Calculated “relative” wind chill temperature, degrees Celsius, to the nearest 0.1 degree\n<3> C = degrees C\n<4> WCHR (ID indicating relative wind chill)\n<5> C = temperature\n<6> Calculated “theoretical” wind chill temperature, degrees Celsius, to the nearest 0.1 degree\n<7> C = degrees C\n<8> WCHT (ID indicating theoretical wind chill)\n<9> C = temperature\n<10> Calculated heat index, degrees Celsius, to the nearest 0.1 degree (this field left blank by WeatherStation)\n<11> C = degrees C\n<12> HINX (ID indicating heat index)\n<13> P = pressure\n<14> Actual measured barometric pressure, or \"station pressure\", bars, to the nearest 0.001 bar\n<15> B = bars\n<16> STNP (ID indicating station pressure)"
          n117 = Fract/Exp String To Number(string=w1171) -> (number=w1167:dbl)  [unwired: 3 in, 1 out]
          n118 = Fract/Exp String To Number(string=w1170) -> (number=w1166:dbl)  [unwired: 3 in, 1 out]
          n119 = Fract/Exp String To Number(string=w1168) -> (number=w1165:dbl)  [unwired: 3 in, 1 out]
          n120 = Fract/Exp String To Number(string=w1169) -> (number=w1164:dbl)  [unwired: 3 in, 1 out]
          n121 = Bundle By Name(cluster=T9 {"Calc. Relative Wind Chill (degC)"=0.0, "Calc. Theoretical Wind Chill (degC)"=0.0, "Calc. Heat Index (degC)"=0.0, "Meas. Barometric Pressure (bars)"=0.0} ("Transducer (XDR) A Data 2"), "Calc. Relative Wind Chill (degC)"=w1167, "Calc. Theoretical Wind Chill (degC)"=w1166, "Calc. Heat Index (degC)"=w1165, "Meas. Barometric Pressure (bars)"=w1164) -> (→"Transducer (XDR) A Data":T9)
        }
      }
    }
  }
